vi "Read_All_Motor_Positions.vi"(6 "Echo Mode":i32, 8 "error in":errorcluster={"status"=FALSE, "code"=1073676294, "source"="VISA Read in write_read.vi"}, 10 "Pos Unit":T1=1 items=["STEPS", "MICRONS / DEG", "MILLIMETER / DEG", "CENTIMETER / DEG", "INCHES / DEG"], 11 "VISA resource name":refnum<visa-resource-name>) -> (0 "error out":errorcluster={"status"=FALSE, "code"=1073676294, "source"="VISA Read in write_read.vi"}, 1 "Manipulator Pos (Steps)":i32[](array[numeric]), 2 "Manipulator Pos (Pos Unit Input)":dbl[](array[numeric]), 3 "VISA out":refnum<visa-resource-name>, 4 "Manipulator Pos (Microns/Degrees)":dbl[](array[numeric]))   [LabVIEW 2018]
uses:
  Units_of_Move.ctl
  ConversionAndInformation/Unit_Control.ctl
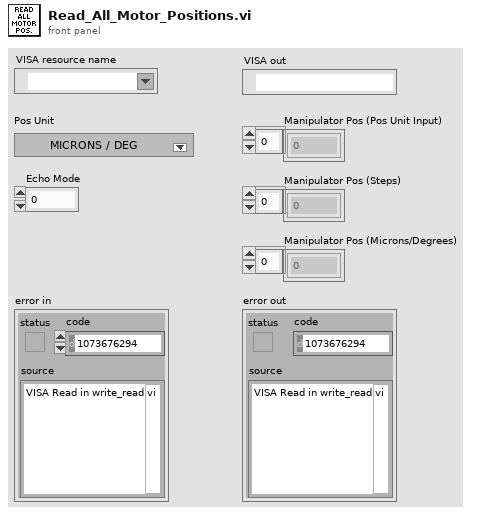
[diagram p1: front panel]
types:
  T1 = typedef "Units_of_Move.ctl" = u16
  T2 = typedef "Unit_Control.ctl" = enum16{"Angle (Degrees)", "Rad", "Angle [TMC]", "Microsteps [TMC]", "Inches", "Nanometer", "Meter", "Centimeter", "Millimeter", "Micron"}
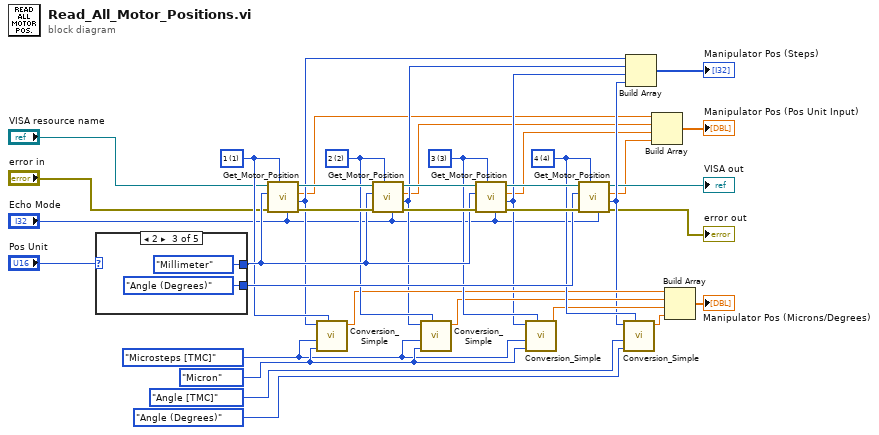
[diagram p0: block diagram]
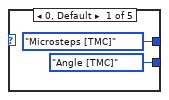
[diagram p2: hidden frame]
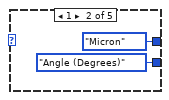
[diagram p3: hidden frame]
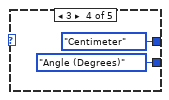
[diagram p4: hidden frame]
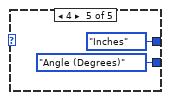
[diagram p5: hidden frame]
diagram:
  w21 = Unit_Control."Micron" ("Input Unit")
  w20 = Unit_Control."Microsteps [TMC]" ("Input Unit")
  w26 = u16 4 items=["none", "1", "2", "3", "4", "all"] ("Motor In")
  w27 = u16 3 items=["none", "1", "2", "3", "4", "all"] ("Motor In")
  w28 = u16 2 items=["none", "1", "2", "3", "4", "all"] ("Motor In")
  w29 = u16 1 items=["none", "1", "2", "3", "4", "all"] ("Motor In")
  n1 = case shown="2" "Pos Unit" {
    tunnel: [Unit_Control."Microsteps [TMC]" ("Output Unit") Unit_Control."Micron" ("Output Unit") Unit_Control."Millimeter" ("Output Unit") Unit_Control."Centimeter" ("Output Unit") Unit_Control."Inches" ("Output Unit")] -> w31
    tunnel: [Unit_Control."Angle [TMC]" ("Output Unit") Unit_Control."Angle (Degrees)" ("Output Unit") Unit_Control."Angle (Degrees)" ("Output Unit") Unit_Control."Angle (Degrees)" ("Output Unit") Unit_Control."Angle (Degrees)" ("Output Unit")] -> w30
    frame 0, Default {
    }
    frame 1 {
    }
    frame 2 {
    }
    frame 3 {
    }
    frame 4 {
    }
  }
  n2 = call "Get_Motor_Position.vi"("Echo Mode (2)"="Echo Mode", "Motor In"=w29, "error in (no error)"="error in", "Output Unit"=w31, "VISA resource name"="VISA resource name") -> ("error out"=w36:errorcluster, "Position (Steps)"=w16:i32, "Position"=w9:dbl, "VISA ressource out"=w37:refnum<visa-resource-name>)  [unwired: 3 in]
  n3 = call "Conversion_Simple.vi"("Motor"=w29, "Output Unit"=w21, "Input Unit"=w20, "Input"=w16) -> ("Output"=w19:dbl)  [unwired: 6 in, 1 out]
  n4 = call "Get_Motor_Position.vi"("Echo Mode (2)"="Echo Mode", "Motor In"=w28, "error in (no error)"=w36, "Output Unit"=w31, "VISA resource name"=w37) -> ("error out"=w33:errorcluster, "Position (Steps)"=w15:i32, "Position"=w8:dbl, "VISA ressource out"=w35:refnum<visa-resource-name>)  [unwired: 3 in]
  n5 = call "Conversion_Simple.vi"("Motor"=w28, "Output Unit"=w21, "Input Unit"=w20, "Input"=w15) -> ("Output"=w23:dbl)  [unwired: 6 in, 1 out]
  n6 = call "Get_Motor_Position.vi"("Echo Mode (2)"="Echo Mode", "Motor In"=w27, "error in (no error)"=w33, "Output Unit"=w31, "VISA resource name"=w35) -> ("error out"=w32:errorcluster, "Position (Steps)"=w14:i32, "Position"=w7:dbl, "VISA ressource out"=w34:refnum<visa-resource-name>)  [unwired: 3 in]
  n7 = call "Conversion_Simple.vi"("Motor"=w27, "Output Unit"=w21, "Input Unit"=w20, "Input"=w14) -> ("Output"=w18:dbl)  [unwired: 6 in, 1 out]
  n8 = call "Get_Motor_Position.vi"("Echo Mode (2)"="Echo Mode", "Motor In"=w26, "error in (no error)"=w32, "Output Unit"=w30, "VISA resource name"=w34) -> ("error out"=→"error out":errorcluster, "Position (Steps)"=w13:i32, "Position"=w6:dbl, "VISA ressource out"=→"VISA out":refnum<visa-resource-name>)  [unwired: 3 in]
  n9 = call "Conversion_Simple.vi"("Motor"=w26, "Output Unit"=Unit_Control."Angle (Degrees)" ("Input Unit"), "Input Unit"=Unit_Control."Angle [TMC]", "Input"=w13) -> ("Output"=w22:dbl)  [unwired: 6 in, 1 out]
  n10 = Build Array(w16, w15, w14, w13) -> (→"Manipulator Pos (Steps)":i32[])
  n11 = Build Array(w9, w8, w7, w6) -> (→"Manipulator Pos (Pos Unit Input)":dbl[])
  n12 = Build Array(w19, w23, w18, w22) -> (→"Manipulator Pos (Microns/Degrees)":dbl[])
